vi "ImageNotifier.vi"() -> ()   [LabVIEW 2017, in "ImageAcquisitionLibrary.lvlib"]
uses:
  ImageAcquisitionLibrary.lvlib
  Acquisition/AcquireData.ctl
panel:
  in  "Display Notifier":refnum<notifier>
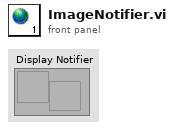
[diagram p1: front panel]
diagram:
